vi "SET ISO BAT MOINS.vi"(8 "Error In":errorcluster, 11 "Port tak":refnum<visa-resource-name>="N/A") -> (0 "Error Out":errorcluster, 3 "UNO TAK out":T1)   [LabVIEW 2020]
uses:
  <vilib>/MakerHub/LINX/Private/Type Defs/LINX Ref.ctl
  <vilib>/MakerHub/LINX/Private/Type Defs/Platform.ctl
  <vilib>/MakerHub/LINX/Private/Type Defs/Interface.ctl
  <vilib>/MakerHub/LINX/Private/Device/Type Defs/LINX Device Config.ctl
  <vilib>/MakerHub/LINX/Private/Device/Type Defs/TCP Config.ctl
  <vilib>/MakerHub/LINX/Private/Device/Type Defs/Channels.ctl
  <vilib>/MakerHub/LINX/Public/Peripherals/Digital/Digital Write 1 Chan.vi
  <vilib>/MakerHub/LINX/Public/Peripherals/Digital/Digital Write N Chans.vi
  <vilib>/MakerHub/LINX/Private/Local IO/LinxDigitalWrite.vi
  <vilib>/MakerHub/LINX/Public/Utilities/Check Channel.vi
  <vilib>/MakerHub/LINX/Public/Utilities/Open Serial.vi
  <vilib>/MakerHub/LINX/Private/Utilties/Generate Error.vi
  <vilib>/MakerHub/LINX/LMH-LINX.lvlib
  <vilib>/MakerHub/LINX/Private/Device/Device.lvlib
panel:
  out "Device Name":string
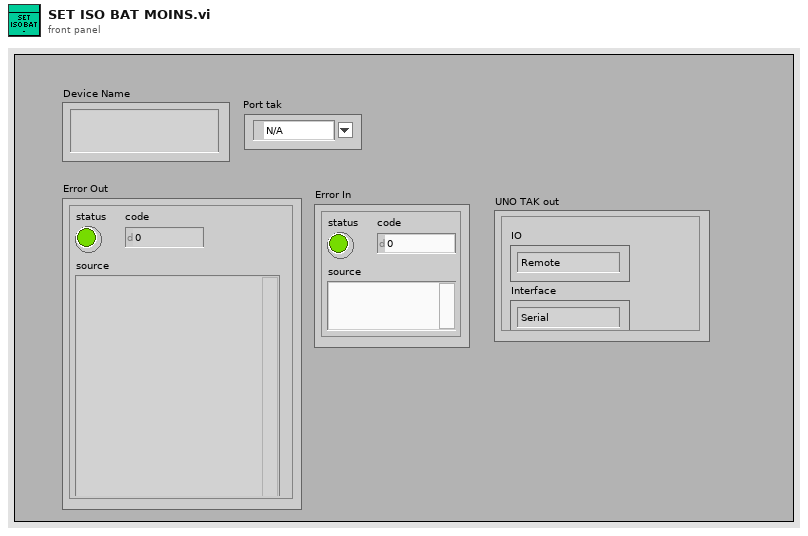
[diagram p1: front panel]
types:
  T1 = typedef "LMH-LINX.lvlib/LINX Ref.ctl" = cluster{"IO":T2, "Interface":T3, "LINX Device Config":T4}
  T2 = typedef "LMH-LINX.lvlib/Platform.ctl" = enum16{"Remote", "Local"}
  T3 = typedef "LMH-LINX.lvlib/Interface.ctl" = enum16{"Serial", "TCP"}
  T4 = typedef "LMH-LINX.lvlib/Device.lvlib/LINX Device Config.ctl" = cluster{"Interface":T3, "COM Port":refnum<visa-resource-name>, "TCP Configuration":T5, "Device Family":u8, "Device ID":u8, "Device Name":string, "TCP Ref":refnum<k5>, "Channels":T6}
  T5 = typedef "LMH-LINX.lvlib/Device.lvlib/TCP Config.ctl" = cluster{"IP Address":string, "Port":u16}
  T6 = typedef "LMH-LINX.lvlib/Channels.ctl" = cluster{"DI":u8[], "DO":u8[], "AI":u8[], "AO":u8[], "PWM":u8[], "QE":u8[], "UART":u8[], "I2C 2":u8[], "SPI":u8[], "CAN":u8[], "Servo":u8[], "AI Ref (V)":dbl, "AI Resolution (Bits)":u8, "AO Ref (V)":dbl, "AO Resolution (Bits)":u8}
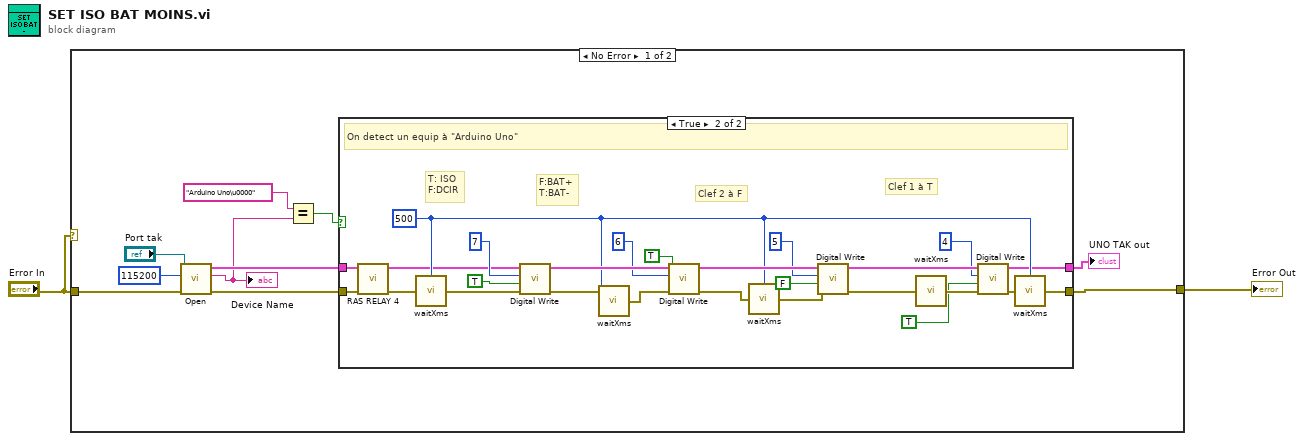
[diagram p0: block diagram]
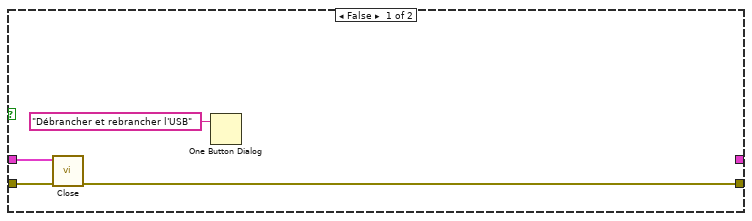
[diagram p2: hidden frame]
diagram:
  n1 = case shown="No Error" "Error In" {
    tunnel: [w5 w43] -> w2
    tunnel: "Error In" -> [w4 w43]
    frame No Error {
      n2 = call-poly <vilib>:"Open.vi"("Error In"=w4, "Baud Rate Override"=u32 115200 ("Baud Rate (115200)"), "Serial Port"="Port tak") -> ("Error Out"=w11:errorcluster, "Device Name"=w7:string, "LINX Resource"=w10:T1)  [unwired: 6 in]
      "Device Name" <- w7
      n3 = Equal?(x="Arduino Uno\u0000", y=w7) -> (x = y?=w6:bool)
      n4 = case shown="True" w6 {
        tunnel: [_ w20] -> w12
        tunnel: [w13 w21] -> w5
        tunnel: w11 -> [w15 w18]
        tunnel: w10 -> [w14 w19]
        frame False {
          n5 = call <vilib>:"Close.vi"("Error In"=w15, "LINX Resource"=w14) -> ("Error Out"=w13:errorcluster)  [unwired: 9 in]
          n6 = One Button Dialog ("Boîte de dialogue à un bouton")(message="Débrancher et rebrancher l'USB") -> ()  [unwired: 1 in, 1 out]
        }
        frame True {
          w25 = u32 500 ("attente (ms)")
          # "F:BAT+\nT:BAT-"
          # "T: ISO\nF:DCIR"
          # "Clef 1 à T"
          # "Clef 2 à F"
          # "On detect un equip à \"Arduino Uno\""
          n7 = call "RAS RELAY 4.vi"("entrée d'erreur (pas d'erreur)"=w18, "LINX Resource en entrée"=w19) -> ("sortie d'erreur"=w23:errorcluster, "LINX Resource en sortie"=w17:T1)  [unwired: 8 in]
          n8 = call <userlib>:"waitXms.vi"("attente (ms)"=w25, "errin"=w23) -> ("errout"=w37:errorcluster)  [unwired: 13 in]
          n9 = call-poly <vilib>:"Digital Write.vi"("Error In"=w37, "Output Value"=TRUE, "DO Channel"=u8 7, "LINX Resource"=w17) -> ("Error Out"=w29:errorcluster, "LINX Resource"=w41:T1)  [unwired: 6 in]
          n10 = call <userlib>:"waitXms.vi"("attente (ms)"=w25, "errin"=w29) -> ("errout"=w28:errorcluster)  [unwired: 13 in]
          n11 = call-poly <vilib>:"Digital Write.vi"("Error In"=w28, "Output Value"=TRUE, "DO Channel"=u8 6, "LINX Resource"=w41) -> ("Error Out"=w27:errorcluster, "LINX Resource"=w39:T1)  [unwired: 6 in]
          n12 = call <userlib>:"waitXms.vi"("attente (ms)"=w25, "errin"=w27) -> ("errout"=w26:errorcluster)  [unwired: 13 in]
          n13 = call-poly <vilib>:"Digital Write.vi"("Error In"=w26, "Output Value"=FALSE, "DO Channel"=u8 5, "LINX Resource"=w39) -> ("Error Out"=w36:errorcluster, "LINX Resource"=w34:T1)  [unwired: 6 in]
          n14 = call <userlib>:"waitXms.vi"("errin"=w36) -> ("errout"=w35:errorcluster)  [unwired: 14 in]
          n15 = call-poly <vilib>:"Digital Write.vi"("Error In"=w35, "Output Value"=TRUE, "DO Channel"=u8 4, "LINX Resource"=w34) -> ("Error Out"=w31:errorcluster, "LINX Resource"=w20:T1)  [unwired: 6 in]
          n16 = call <userlib>:"waitXms.vi"("attente (ms)"=w25, "errin"=w31) -> ("errout"=w21:errorcluster)  [unwired: 13 in]
        }
      }
      "UNO TAK out" <- w12
    }
    frame Error {
    }
  }
  "Error Out" <- w2
